vi "Facade 1.vi"(0 "Data In":T4, 2 "Display State In":T2, 3 "Container State":T3) -> (6 "Data Out":T4, 7 "Display State Out":T2, 8 "Action":T1)   [LabVIEW 2021, in "管路電子閥.xctl"]
uses:
  Data 1.ctl
  <vilib>/_xctls/Container State.ctl
  State 1.ctl
  <vilib>/_xctls/Action.ctl
  <vilib>/_xctls/XControlSupport.lvlib
panel:
  in  "開關":bool
  in  "圖片未啟動":path
  in  "圖片啟動":path
  out "顯示圖片":picture
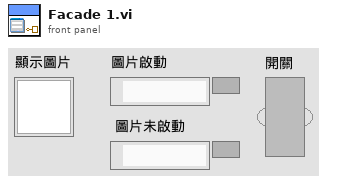
[diagram p1: front panel]
types:
  T1 = typedef "XControlSupport.lvlib/Action.ctl" = cluster{"Data Changed?":bool, "State Changed?":bool, "Action Name":string}
  T2 = typedef "管路電子閥.xctl/State 1.ctl" = cluster{"Numeric":dbl}
  T3 = typedef "XControlSupport.lvlib/Container State.ctl" = cluster{"Indicator?":bool, "Run Mode?":bool, " Refnum":refnum<vi>}
  T4 = typedef "管路電子閥.xctl/Data 1.ctl" = bool
  T5 = typedef "imagedata.ctl" = cluster{"image type":i32, "image depth":i32, "image":u8[], "mask":u8[], "colors":u32[], "Rectangle":cluster{"left":i16, "top":i16, "right":i16, "bottom":i16}}
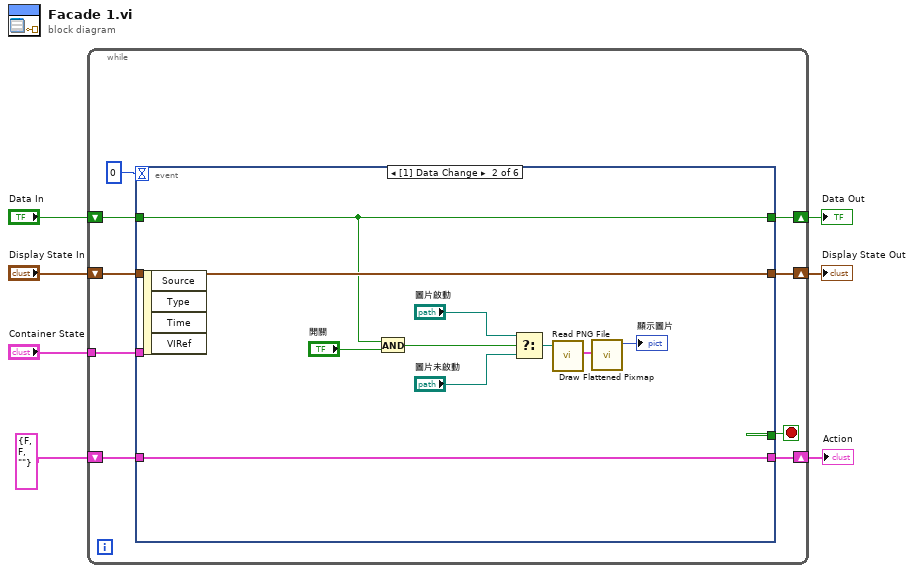
[diagram p0: block diagram]
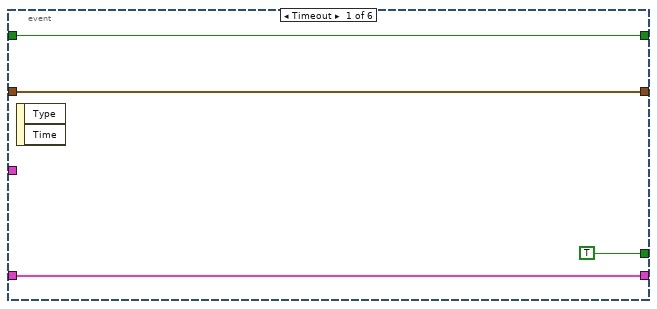
[diagram p2: hidden frame]
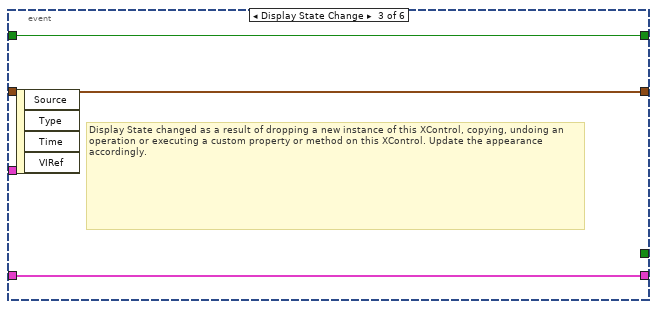
[diagram p3: hidden frame]
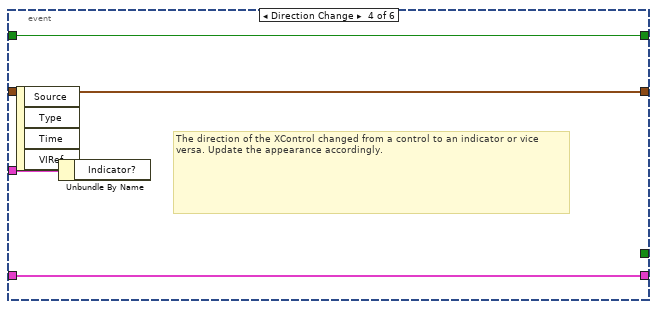
[diagram p4: hidden frame]
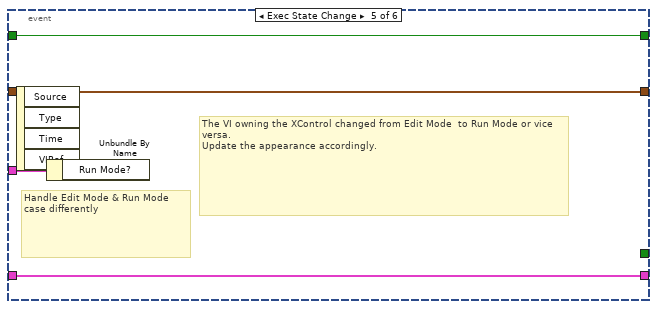
[diagram p5: hidden frame]
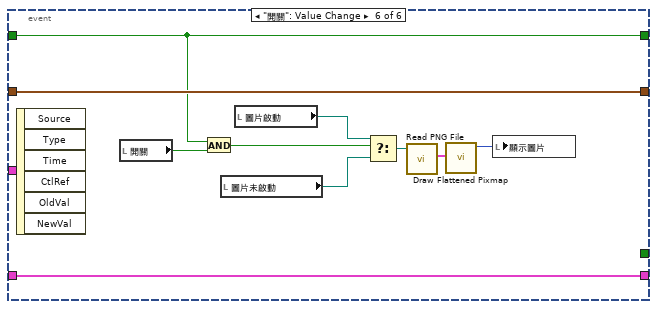
[diagram p6: hidden frame]
diagram:
  n1 = while {
    shift-right: [w15] -> w4
    shift-left: "Display State In" -> [w16]
    tunnel: "Container State" -> [w12]
    shift-right: [w10] -> w7
    shift-left: "Data In" -> [w11]
    shift-right: [w8] -> w2
    shift-left: T1 {"Data Changed?"=FALSE, "State Changed?"=FALSE, "Action Name"=""} ("Action") -> [w9]
    stop <- w14 stop-if-true
    n2 = event shown="[1] Data Change" {
      selector: _ -> [_ _ _ _ _ _]
      dyn-events: _ -> [_ _ _ _ _ _]
      timeout: 0 -> [_ _ _ _ _ _]
      tunnel: w16 -> [w18 w30 w33 w36 w40 w51]
      tunnel: [w18 w30 w33 w36 w40 w51] -> w15
      tunnel: [TRUE _ _ _ _ _] -> w14
      tunnel: w12 -> [_ _ _ w37 w41 _]
      tunnel: w11 -> [w17 w22 w32 w35 w39 w43]
      tunnel: [w17 w22 w32 w35 w39 w43] -> w10
      tunnel: [w19 w29 w31 w34 w38 w50] -> w8
      tunnel: w9 -> [w19 w29 w31 w34 w38 w50]
      event Timeout {
        n3 = event-data() -> ()  [unwired: 1 in, 2 out]
      }
      event Data Change {
        n4 = event-data() -> ()  [unwired: 1 in, 4 out]
        n5 = And(x=w22, y="開關") -> (x .and. y?=w23:T4)
        n6 = Select(t="圖片啟動", s=w23, f="圖片未啟動") -> (s? t:f=w26:path)
        n7 = call <vilib>:"Read PNG File.vi"("path to PNG file"=w26) -> ("image data"=w28:T5)  [unwired: 8 in, 2 out]
        n8 = call <vilib>:"Draw Flattened Pixmap.vi"("image data"=w28) -> ("new picture"=→"顯示圖片":picture)  [unwired: 8 in]
      }
      event Display State Change {
        # "Display State changed as a result of dropping a new instance of this XControl, copying, undoing an operation or executing a custom property or method on this XControl. Update the appearance accordingly."
        n9 = event-data() -> ()  [unwired: 1 in, 4 out]
      }
      event Direction Change {
        # "The direction of the XControl changed from a control to an indicator or vice versa. Update the appearance accordingly."
        n10 = event-data() -> ()  [unwired: 1 in, 4 out]
        n11 = Unbundle By Name(w37) -> ()  [unwired: 1 out]
      }
      event Exec State Change {
        # "The VI owning the XControl changed from Edit Mode  to Run Mode or vice versa.\nUpdate the appearance accordingly."
        # "Handle Edit Mode & Run Mode\ncase differently"
        n12 = event-data() -> ()  [unwired: 1 in, 4 out]
        n13 = Unbundle By Name(w41) -> ()  [unwired: 1 out]
      }
      event "開關": Value Change {
        n14 = event-data() -> ()  [unwired: 1 in, 6 out]
        n15 = local read "開關"() -> (w42:bool)
        n16 = And(x=w43, y=w42) -> (x .and. y?=w44:T4)
        n17 = local read "圖片未啟動"() -> (w45:path)
        n18 = local read "圖片啟動"() -> (w46:path)
        n19 = Select(t=w46, s=w44, f=w45) -> (s? t:f=w48:path)
        n20 = call <vilib>:"Read PNG File.vi"("path to PNG file"=w48) -> ("image data"=w49:T5)  [unwired: 8 in, 2 out]
        n21 = call <vilib>:"Draw Flattened Pixmap.vi"("image data"=w49) -> ("new picture"=w47:picture)  [unwired: 8 in]
        n22 = local write "顯示圖片"(w47) -> ()
      }
    }
  }
  "Display State Out" <- w4
  "Data Out" <- w7
  "Action" <- w2
